vi "Change DC Offset Voltage.vi"(8 "error in (no error)":errorcluster, 10 "DC Offset":dbl, 11 "Device in":refnum<class "Device.lvclass">) -> (0 "error out":errorcluster, 3 "Device out":refnum<class "Device.lvclass">)   [LabVIEW 2020, in "Device.lvclass"]
uses:
  Device.lvclass
  Instruments/Power Supply/Power Supply.lvclass
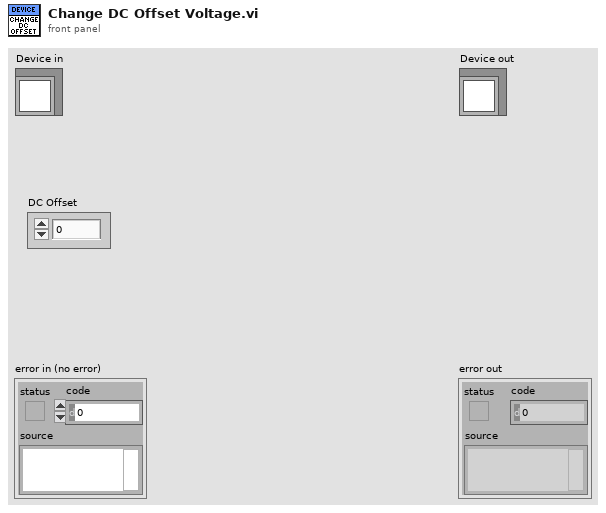
[diagram p1: front panel]
types:
  T1 = typedef "Device.lvclass/DC Offset Cluster.ctl" = cluster{"Enable":bool, "Use Array":bool, "Array":dbl[], "To From Cluster":cluster{"From":dbl, "To":dbl, "Step":dbl}, "Current Value":dbl, "DC Offset":refnum<class "Power Supply.lvclass">}
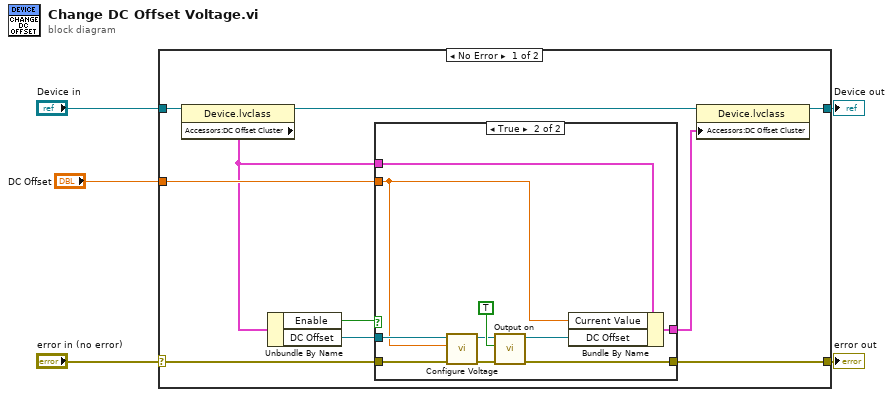
[diagram p0: block diagram]
diagram:
  n1 = case shown="No Error" "error in (no error)" {
    selector: "error in (no error)" -> [w12 w29]
    tunnel: [w10 w29] -> w4
    tunnel: [w9 w28] -> w2
    tunnel: "Device in" -> [w15 w28]
    tunnel: "DC Offset" -> [w11 _]
    frame No Error {
      n2 = property class="Device.lvclass"(reference=w15) -> (reference out=w7:refnum<class "Device.lvclass">, "Accessors:DC Offset Cluster"=w8:T1)  [unwired: 1 in, 1 out]
      n3 = Unbundle By Name(w8) -> ("Enable"=w14:bool, "DC Offset"=w13:refnum<class "Power Supply.lvclass">)
      n4 = case shown="True" w14 {
        tunnel: w13 -> [_ w26]
        tunnel: w12 -> [w17 w25]
        tunnel: w11 -> [_ w18]
        tunnel: [w17 w23] -> w10
        tunnel: w8 -> [w16 w19]
        tunnel: [w16 w21] -> w6
        frame False {
        }
        frame True {
          n5 = call-dynamic "Configure Voltage.vi"("error in (no error)"=w25, "Voltage"=w18, "Power Supply in"=w26) -> ("error out"=w24:errorcluster, "Power Supply out"=w22:refnum<class "Power Supply.lvclass">)  [unwired: 7 in]
          n6 = call-dynamic "Output on.vi"("error in (no error)"=w24, "Output On"=TRUE, "Power Supply in"=w22) -> ("error out"=w23:errorcluster, "Power Supply out"=w20:refnum<class "Power Supply.lvclass">)  [unwired: 7 in]
          n7 = Bundle By Name(cluster=w19, "Current Value"=w18, "DC Offset"=w20) -> (w21:T1)
        }
      }
      n8 = property class="Device.lvclass"(reference=w7, "Accessors:DC Offset Cluster"=w6) -> (reference out=w9:refnum<class "Device.lvclass">)  [unwired: 1 in, 1 out]
    }
    frame Error {
    }
  }
  "error out" <- w4
  "Device out" <- w2
